vi "Relay Control.vi"(8 "error in (no error)":errorcluster, 9 "relay action (Close Relay)":T1=enum."Close Relay", 10 "relay string":string, 11 "SLSC Switch in":refnum<class "SLSC Switch.lvclass">) -> (0 "error out":errorcluster, 3 "SLSC Switch out":refnum<class "SLSC Switch.lvclass">)   [LabVIEW 2015, in "SLSC Switch.lvclass"]
uses:
  SLSC Switch.lvclass
  slscsl/RelayAction.ctl
  slscsl/slscsl.lvclass
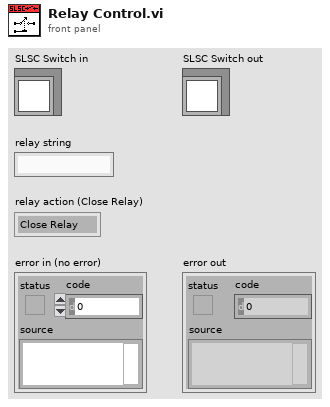
[diagram p1: front panel]
types:
  T1 = typedef "slscsl.lvclass/RelayAction.ctl" = enum16{"Open Relay", "Close Relay"}
  T2 = typedef "SLSC Switch.lvclass/SLSC Relay Info.ctl" = cluster{"physicalChannel":T3, "property":refnum<k21>, "command":refnum<k21>}
  T3 = typedef "SLSC Switch.lvclass/Physical Channel.ctl" = cluster{"name":refnum<k21>, "property":refnum<k21>}
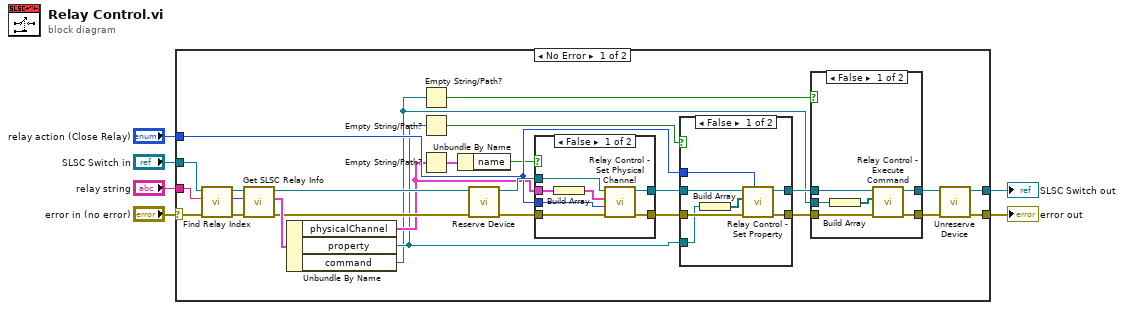
[diagram p0: block diagram]
diagram:
  n1 = case shown="No Error" "error in (no error)" {
    selector: "error in (no error)" -> [w23 w61]
    tunnel: [w25 w61] -> w5
    tunnel: [w27 w60] -> w3
    tunnel: "SLSC Switch in" -> [w24 w60]
    tunnel: "relay action (Close Relay)" -> [w17 _]
    tunnel: "relay string" -> [w19 _]
    frame No Error {
      n2 = call "Find Relay Index.vi"("error in (no error)"=w23, "relay string"=w19, "SLSC Switch in"=w24) -> ("error out"=w22:errorcluster, "index"=w21:i32, "SLSC Switch out"=w20:refnum<class "SLSC Switch.lvclass">)  [unwired: 6 in]
      n3 = call "Get SLSC Relay Info.vi"("error in (no error)"=w22, "relay index"=w21, "SLSC Switch in"=w20) -> ("error out"=w26:errorcluster, "SLSC Switch Info"=w33:T2, "SLSC Switch out"=w30:refnum<class "SLSC Switch.lvclass">)  [unwired: 6 in]
      n4 = Unbundle By Name(w33) -> ("physicalChannel"=w13:T3, "property"=w9:refnum<k21>, "command"=w8:refnum<k21>)
      n5 = Empty String/Path?(string/path=w8) -> (empty?=w7:bool)
      n6 = Empty String/Path?(string/path=w9) -> (empty?=w10:bool)
      n7 = Empty String/Path?(string/path=w13) -> (empty?=w12:cluster{"name":bool, "property":bool})
      n8 = Unbundle By Name(w12) -> ("name"=w11:bool)
      n9 = call "Reserve Device.vi"("error in (no error)"=w26, "SLSC Switch in"=w30) -> ("error out"=w16:errorcluster, "SLSC Switch out"=w18:refnum<class "SLSC Switch.lvclass">)  [unwired: 8 in]
      n10 = case shown="False" w11 {
        tunnel: w18 -> [w57 w59]
        tunnel: w17 -> [w55 _]
        tunnel: w16 -> [w54 w58]
        tunnel: [w53 w58] -> w15
        tunnel: [w52 w59] -> w14
        tunnel: w13 -> [w51 _]
        frame False {
          n11 = Build Array(w51) -> (w56:T3[])
          n12 = call "Relay Control - Set Physical Channel.vi"("error in (no error)"=w54, "relay action (Close Relay)"=w55, "Physical Channels"=w56, "SLSC Switch in"=w57) -> ("error out"=w53:errorcluster, "SLSC Switch out"=w52:refnum<class "SLSC Switch.lvclass">)  [unwired: 6 in]
        }
        frame True {
        }
      }
      n13 = case shown="False" w10 {
        tunnel: [w48 w49] -> w32
        tunnel: [w47 w50] -> w29
        tunnel: w17 -> [w46 _]
        tunnel: w15 -> [w45 w49]
        tunnel: w14 -> [w44 w50]
        tunnel: w9 -> [w42 _]
        frame False {
          n14 = Build Array(w42) -> (w43:refnum<k21>[])
          n15 = call "Relay Control - Set Property.vi"("relay action (Close Relay)"=w46, "error in (no error)"=w45, "Properties"=w43, "SLSC Switch in"=w44) -> ("error out"=w48:errorcluster, "SLSC Switch out"=w47:refnum<class "SLSC Switch.lvclass">)  [unwired: 6 in]
        }
        frame True {
        }
      }
      n16 = case shown="False" w7 {
        tunnel: w32 -> [w39 w40]
        tunnel: [w38 w40] -> w31
        tunnel: w29 -> [w37 w41]
        tunnel: [w36 w41] -> w28
        tunnel: w8 -> [w35 _]
        frame False {
          n17 = Build Array(w35) -> (w34:refnum<k21>[])
          n18 = call "Relay Control - Execute Command.vi"("error in (no error)"=w39, "Commands"=w34, "SLSC Switch in"=w37) -> ("error out"=w38:errorcluster, "SLSC Switch out"=w36:refnum<class "SLSC Switch.lvclass">)  [unwired: 7 in]
        }
        frame True {
        }
      }
      n19 = call "Unreserve Device.vi"("error in (no error)"=w31, "SLSC Switch in"=w28) -> ("error out"=w25:errorcluster, "SLSC Switch out"=w27:refnum<class "SLSC Switch.lvclass">)  [unwired: 8 in]
    }
    frame Error {
    }
  }
  "error out" <- w5
  "SLSC Switch out" <- w3
